vi "TEMPLATE.vi"(6 "Teller":refnum<class "Teller.lvclass">, 11 "TEMPLATE in":refnum<class "TEMPLATE.lvclass">) -> (0 "Error out":errorcluster, 3 "TEMPLATE out":refnum<class "TEMPLATE.lvclass">)   [LabVIEW 2025, in "_Template.lvlib" / "Templates.lvlib" / "TEMPLATE Msg.lvlib" / "TEMPLATE.lvclass"]
uses:
  TEMPLATE.lvclass
  jettl/jettl/Teller/Teller.lvclass
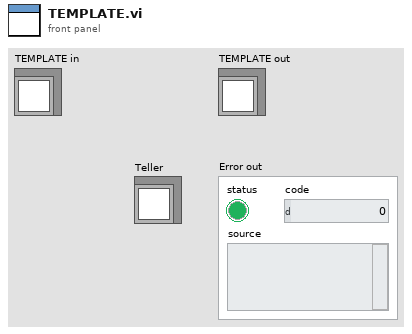
[diagram p1: front panel]
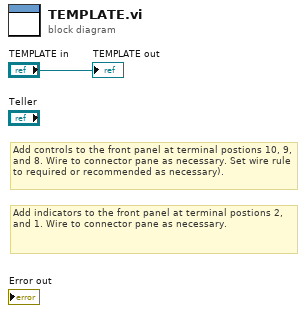
[diagram p0: block diagram]
diagram:
  # "Add indicators to the front panel at terminal postions 2, and 1. Wire to connector pane as necessary."
  # "Add controls to the front panel at terminal postions 10, 9, and 8. Wire to connector pane as necessary. Set wire rule to required or recommended as necessary)."
  "TEMPLATE out" <- "TEMPLATE in"
